vi "ZieglerNichols.vi"(6 "Pc":dbl, 7 "Kc":dbl) -> (1 "Kd":dbl, 2 "Ki":dbl, 3 "Kp":dbl)   [LabVIEW 2015]
doc: "Produces PID coefficients using the Ziegler-Nichols method."
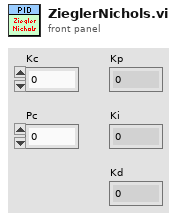
[diagram p1: front panel]
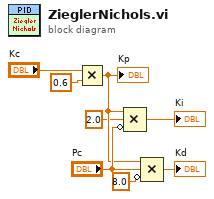
[diagram p0: block diagram]
diagram:
  n1 = Multiply(x="Kc", y=0.6) -> (x*y=w4:dbl)
  "Kp" <- w4
  n2 = Compound Arithmetic op=MULTIPLY(w4, 2.0 ("value"), invert "Pc") -> (→"Ki":dbl)
  n3 = Compound Arithmetic op=MULTIPLY(w4, "Pc", invert 8.0 ("value")) -> (→"Kd":dbl)
